vi "Deploy to Resource.vi"(8 "error in (no error)":errorcluster, 9 "Resource":refnum<class "DeployResource.lvclass">, 10 "VIA":string, 11 "RP2040Target in":refnum<class "RP2040Target.lvclass">) -> (0 "error out":errorcluster, 2 "Response":string, 3 "RP2040Target out":refnum<class "RP2040Target.lvclass">)   [LabVIEW 2020, in "RP2040.lvlib" / "RP2040Target.lvclass"]
uses:
  RP2040Target.lvclass
  Builds/picoG/ppl/PicoG-Core.lvlibp/DeployResource/DeployResource.lvclass
  VisaResource/VisaResource.lvclass
  1caef962-1e4a-46d8-8105-61d220e49f3d.vi
  2555fd0a-863b-486f-a404-2a7442b3f8ba.vi
  <vilib>/Instr/_visa.llb/VISA Configure Serial Port (Instr).vi
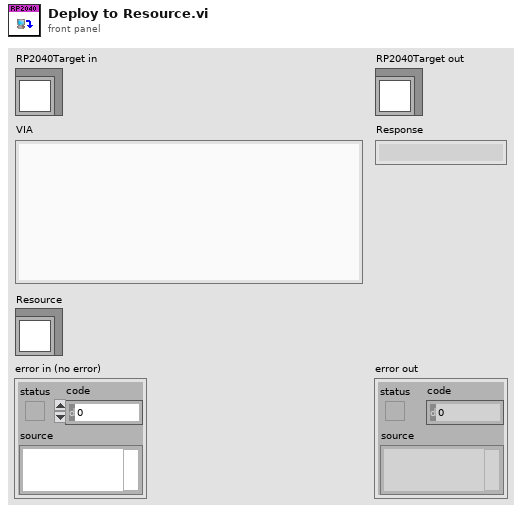
[diagram p1: front panel]
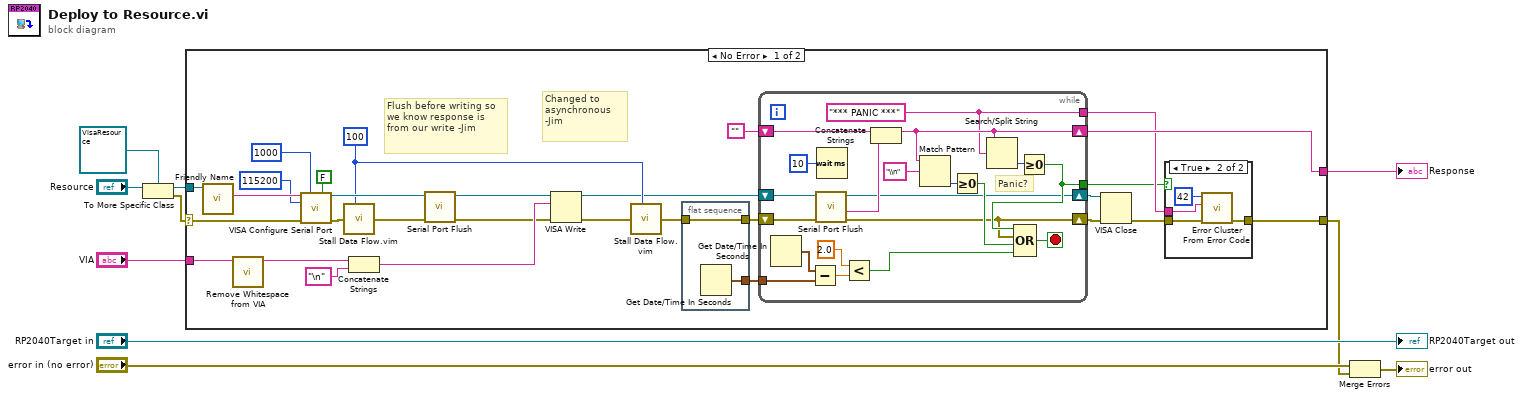
[diagram p0: block diagram]
diagram:
  n1 = To More Specific Class(target class=refnum<class "VisaResource.lvclass"> refnum ("RP2040.lvlib:VisaResource"), reference="Resource") -> (specific class reference=w6:refnum<class "VisaResource.lvclass">, error out=w5:errorcluster)  [unwired: 1 in]
  n2 = case shown="No Error" w5 {
    selector: w5 -> [w31 w67]
    tunnel: w6 -> [w39 _]
    tunnel: [w15 w67] -> w1
    tunnel: "VIA" -> [w29 _]
    tunnel: [w25 _] -> w3
    frame No Error {
      w16 = u32 100 ("milliseconds to wait")
      # "Changed to asynchronous -Jim"
      # "Flush before writing so we know response is from our write -Jim"
      n3 = call-dynamic "Friendly Name.vi"("VisaResource in"=w39) -> ("Friendly Name"=w38:string)  [unwired: 8 in, 2 out]
      n4 = call "Remove Whitespace from VIA.vi"("Pretty Printed VIA"=w29) -> ("Ugly Printed VIA"=w28:string)  [unwired: 10 in]
      n5 = call-poly "VISA Configure Serial Port"("VISA resource name"=w38, "timeout (10sec)"=u32 1000, "Enable Termination\nChar (T)"=FALSE ("Enable Termination\nChar (T)"), "baud rate (9600)"=u32 115200, "error in (no error)"=w31) -> ("VISA resource name out"=w21:refnum<visa-resource-name>, "error out"=w36:errorcluster)  [unwired: 9 in]
      n6 = call "Stall Data Flow.vim"("value in"=w36, "milliseconds to wait"=w16) -> ("value out"=w20:errorcluster)  [unwired: 1 out]
      n7 = Concatenate Strings(w28, "\n" ("string")) -> (w19:string)
      n8 = call "Serial Port Flush.vi"("error in (no error)"=w20, "VISA resource name"=w21) -> ("error out"=w14:errorcluster, "duplicate VISA resource name"=w12:refnum<visa-resource-name>)  [unwired: 7 in, 1 out]
      n9 = VISA Write(VISA resource name=w12, write buffer=w19, error in (no error)=w14) -> (VISA resource name out=w11:refnum<visa-resource-name>, error out=w13:errorcluster)  [unwired: 1 out]
      n10 = call "Stall Data Flow.vim"("value in"=w13, "milliseconds to wait"=w16) -> ("value out"=w17:errorcluster)  [unwired: 1 out]
      n11 = flat-sequence {
        tunnel: w17 -> [w41]
        tunnel: [w41] -> w18
        tunnel: [w40] -> w34
        frame #0 {
          n12 = Get Date/Time In Seconds() -> (seconds since 1Jan1904=w40:timestamp)
        }
      }
      n13 = while {
        shift-right: [w42] -> w33
        shift-left: w18 -> [w45]
        shift-right: [w43] -> w32
        shift-left: w11 -> [w46]
        tunnel: w34 -> [w61]
        shift-right: [w50] -> w25
        shift-left: "" -> [w54]
        tunnel: [w48] -> w23
        tunnel: [w47] -> w22
        stop <- w57 stop-if-true
        w48 = "*** PANIC ***" ("regular expression")
        # "Panic?"
        n14 = Get Date/Time In Seconds() -> (seconds since 1Jan1904=w60:timestamp)
        n15 = Subtract(x=w60, y=w61) -> (x-y=w59:dbl)
        n16 = call "Serial Port Flush.vi"("error in (no error)"=w45, "VISA resource name"=w46) -> ("error out"=w42:errorcluster, "FLUSHED CHARS"=w44:string, "duplicate VISA resource name"=w43:refnum<visa-resource-name>)  [unwired: 7 in]
        n17 = Wait (ms)(milliseconds to wait=u32 10) -> ()  [unwired: 1 out]
        n18 = Less?(x=2.0, y=w59) -> (x < y?=w56:bool)
        n19 = Concatenate Strings(w54, w44) -> (w50:string)
        n20 = Match Pattern(string=w50, regular expression="\\n") -> (offset past match=w52:i32)  [unwired: 1 in, 3 out]
        n21 = Greater Or Equal To 0?(x=w52) -> (x >= 0?=w51:bool)
        n22 = Search/Split String(string=w50, search string/char (-)=w48) -> (offset of match=w49:i32)  [unwired: 1 in, 2 out]
        n23 = Greater Or Equal To 0?(x=w49) -> (x >= 0?=w47:bool)
        n24 = Compound Arithmetic op=OR(w47, w42, w51, w56) -> (w57:bool)
      }
      n25 = VISA Close(VISA resource name=w32, error in (no error)=w33) -> (error out=w24:errorcluster)
      n26 = case shown="True" w22 {
        tunnel: w24 -> [w62 w65]
        tunnel: [w62 w64] -> w15
        tunnel: w23 -> [_ w63]
        frame False {
        }
        frame True {
          n27 = call <vilib>:"Error Cluster From Error Code.vi"("error in (no error)"=w65, "error message (\"\")"=w63, "error code (0)"=42) -> ("error out"=w64:errorcluster)  [unwired: 6 in]
        }
      }
    }
    frame Error {
    }
  }
  "Response" <- w3
  n28 = Merge Errors("error in (no error)", w1) -> (→"error out":errorcluster)
  "RP2040Target out" <- "RP2040Target in"
